vi "DSF.Engine.Transceiver.Shutdown.vi"(8 "error in (no error)":errorcluster, 11 "PXImc Transceiver in":refnum<class "DSF.Transceiver.PXImc.lvclass">) -> (0 "error out":errorcluster, 3 "PXImc Transceiver out":refnum<class "DSF.Transceiver.PXImc.lvclass">)   [LabVIEW 2018, in "DSF.Transceiver.PXImc.lvlib" / "DSF.Transceiver.PXImc.lvclass"]
uses:
  DSF.Transceiver.PXImc.lvclass
  DSF.Transceiver.PXImc.lvclass/DSF.Transceiver.PXImc.ctl
  <vilib>/pximc/nipximc.lvlib
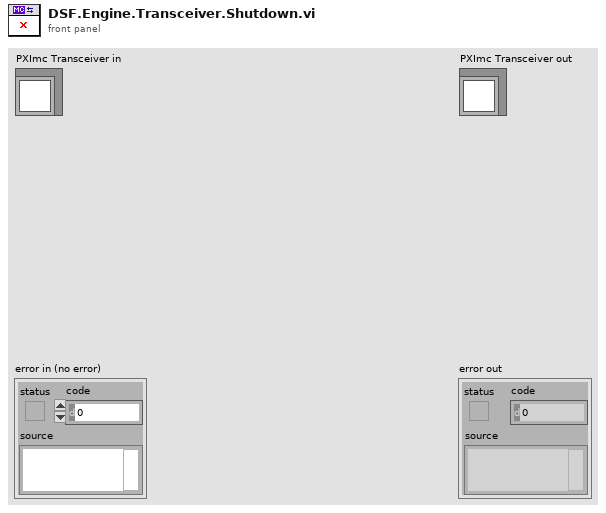
[diagram p1: front panel]
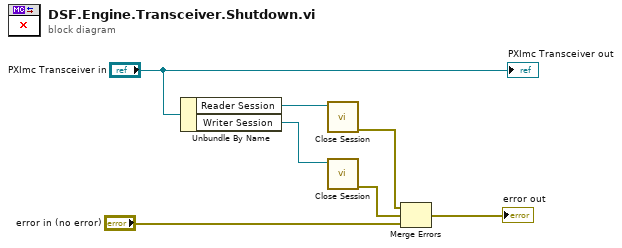
[diagram p0: block diagram]
diagram:
  n1 = Unbundle By Name("PXImc Transceiver in") -> ("Reader Session"=w6:refnum<k21>, "Writer Session"=w5:refnum<k21>)
  n2 = call <vilib>:"Close Session.vi"("session in"=w6) -> ("error out"=w4:errorcluster)  [unwired: 10 in]
  n3 = call <vilib>:"Close Session.vi"("session in"=w5) -> ("error out"=w3:errorcluster)  [unwired: 10 in]
  n4 = Merge Errors(w4, w3, "error in (no error)") -> (→"error out":errorcluster)
  "PXImc Transceiver out" <- "PXImc Transceiver in"
